vi "device.vi"() -> ()   [LabVIEW 2018]
uses:
  <vilib>/MediaMongrels Ltd/WebSockets/WebSockets/WebSocket Client/WebSocket Client.lvclass
  D:/software_setup/National Instruments/LabVIEW 2018/vi.lib/MediaMongrels Ltd/WebSockets/WebSockets/WebSocket/WebSocket.lvclass
panel:
  out "result-GetDeviceName":string
  out "result-GetDeviceVersion":string
  out "result-GetHardwareVersion":string
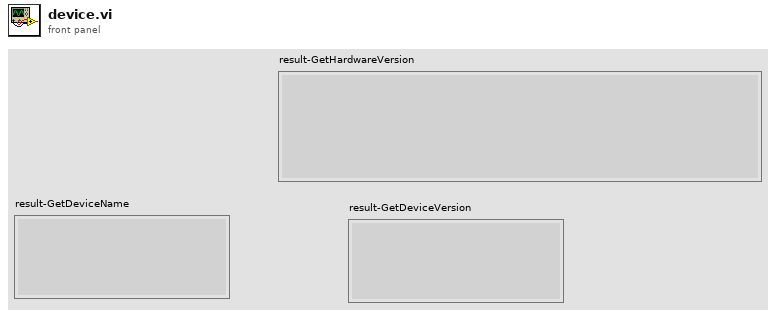
[diagram p1: front panel]
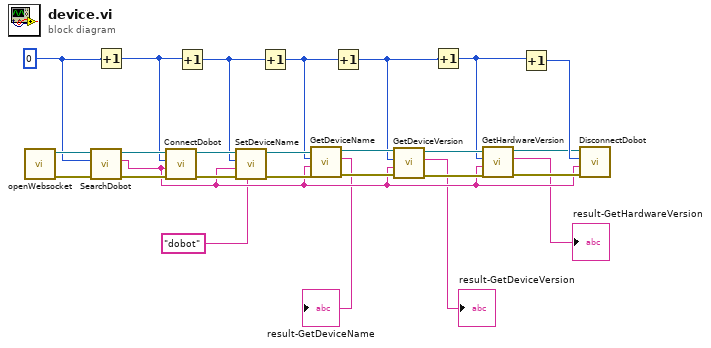
[diagram p0: block diagram]
diagram:
  w22 = 0 ("id")
  n1 = call <vilib>:"openWebsocket.vi"() -> ("error out"=w24:errorcluster, "WebSocket Client out"=w26:refnum<class "WebSocket Client.lvclass">)  [unwired: 10 in]
  n2 = call <vilib>:"SearchDobot.vi"("error in (no error)"=w24, "id"=w22, "WebSocket in"=w26) -> ("error out"=w23:errorcluster, "portName"=w5:string, "WebSocket out"=w25:refnum<class "WebSocket Client.lvclass">)  [unwired: 6 in]
  n3 = Increment(x=w22) -> (x+1=w21:i32)
  n4 = call <vilib>:"ConnectDobot.vi"("error in (no error)"=w23, "portName"=w5, "id"=w21, "WebSocket in"=w25) -> ("error out"=w14:errorcluster, "WebSocket out"=w19:refnum<class "WebSocket Client.lvclass">)  [unwired: 5 in, 1 out]
  n5 = Increment(x=w21) -> (x+1=w9:i32)
  n6 = call <vilib>:"SetDeviceName.vi"("deviceName"="dobot", "error in (no error)"=w14, "portName"=w5, "id"=w9, "WebSocket in"=w19) -> ("error out"=w13:errorcluster, "WebSocket out"=w18:refnum<class "WebSocket Client.lvclass">)  [unwired: 4 in, 1 out]
  n7 = Increment(x=w9) -> (x+1=w8:i32)
  n8 = call <vilib>:"GetDeviceName.vi"("error in (no error)"=w13, "portName"=w5, "id"=w8, "WebSocket in"=w18) -> ("error out"=w12:errorcluster, "deviceName"=→"result-GetDeviceName":string, "WebSocket out"=w17:refnum<class "WebSocket Client.lvclass">)  [unwired: 5 in]
  n9 = Increment(x=w8) -> (x+1=w7:i32)
  n10 = call <vilib>:"GetDeviceVersion.vi"("error in (no error)"=w12, "portName"=w5, "id"=w7, "WebSocket in"=w17) -> ("error out"=w11:errorcluster, "Data"=→"result-GetDeviceVersion":string, "WebSocket out"=w16:refnum<class "WebSocket Client.lvclass">)  [unwired: 5 in]
  n11 = Increment(x=w7) -> (x+1=w6:i32)
  n12 = call <vilib>:"GetHardwareVersion.vi"("error in (no error)"=w11, "portName"=w5, "id"=w6, "WebSocket in"=w16) -> ("error out"=w10:errorcluster, "Data"=→"result-GetHardwareVersion":string, "WebSocket out"=w15:refnum<class "WebSocket Client.lvclass">)  [unwired: 5 in]
  n13 = Increment(x=w6) -> (x+1=w20:i32)
  n14 = call <vilib>:"DisconnectDobot.vi"("error in (no error)"=w10, "portName"=w5, "id"=w20, "WebSocket in"=w15) -> ()  [unwired: 5 in, 3 out]
